vi "Stepper ToGo.vi"(8 "error in":errorcluster, 11 "Arduino Resource":T1={"VISA resource"="", "Board Type"=enum."Arduino Uno", "Connection Type"=enum."USB / Serial", "Bytes Per Packet (15)"=15}) -> (0 "error out":errorcluster, 1 "Steps remaining":u16, 2 "Steps Remaining?":bool, 3 "Arduino Resource Out":T1={"VISA resource"="", "Board Type"=enum."Arduino Uno", "Connection Type"=enum."USB / Serial", "Bytes Per Packet (15)"=15})   [LabVIEW 2011, in "LabVIEW Interface for Arduino.lvlib"]
doc: "Check to see if the Arduino is still processing a previous step command. Wait until Steps Remaining? is false to ensure step commands aren't overwritten."
uses:
  <vilib>/LabVIEW Interface for Arduino/LabVIEW Interface for Arduino.lvlib
  <vilib>/LabVIEW Interface for Arduino/Private/Type Defs/Arduino Resource.ctl
  <vilib>/LabVIEW Interface for Arduino/Private/Type Defs/Board Type.ctl
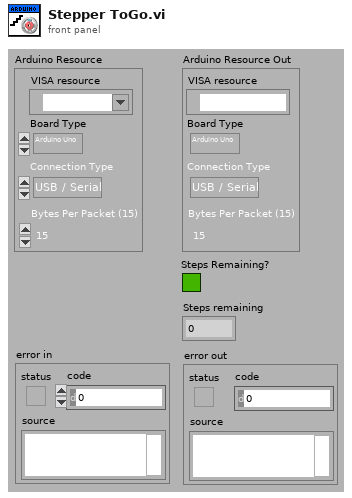
[diagram p1: front panel]
types:
  T1 = typedef "LabVIEW Interface for Arduino.lvlib/Arduino Resource.ctl" = cluster{"VISA resource":refnum<visa-resource-name>, "Board Type":T2, "Connection Type":enum8{"USB / Serial"}, "Bytes Per Packet (15)":u8}
  T2 = typedef "LabVIEW Interface for Arduino.lvlib/Board Type.ctl" = enum16{"Arduino Uno", "Dimuelanove w/Atmega 328", "Mega 2560", "Chipkit Uno32", "Chipkit Max32"}
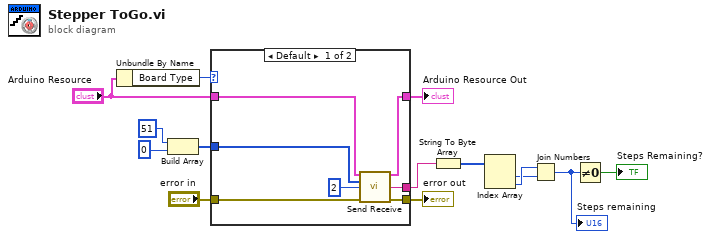
[diagram p0: block diagram]
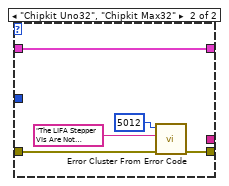
[diagram p2: hidden frame]
diagram:
  n1 = Unbundle By Name("Arduino Resource") -> ("Board Type"=w1:T2)
  n2 = Build Array(u8 51, u8 0 ("element")) -> (w7:u8[])
  n3 = case shown="Default" w1 {
    tunnel: [w19 w24] -> w4
    tunnel: "Arduino Resource" -> [w20 w23]
    tunnel: w7 -> [w18 _]
    tunnel: [w17 w23] -> w6
    tunnel: "error in" -> [w16 w22]
    tunnel: [w15 _] -> w5
    frame Default {
      n4 = call <vilib>:"Send Receive.vi"("Arduino Resource"=w20, "Data"=w18, "Bytes To Read (0)"=u8 2, "error in"=w16) -> ("Arduino Resource"=w17:T1, "Read Buffer"=w15:string, "error out"=w19:errorcluster)  [unwired: 9 in]
    }
    frame "Chipkit Uno32", "Chipkit Max32" {
      n5 = call <vilib>:"Error Cluster From Error Code.vi"("error in (no error)"=w22, "error message (\"\")"="The LIFA Stepper VIs Are Not Supported On Chipkit Targets." ("source"), "error code (0)"=5012) -> ("error out"=w24:errorcluster)  [unwired: 6 in]
    }
  }
  "Arduino Resource Out" <- w6
  "error out" <- w4
  n6 = String To Byte Array(string=w5) -> (unsigned byte array=w13:u8[])
  n7 = Index Array(array=w13) -> (element #1=w10:u8, element #2=w11:u8)  [unwired: 2 in]
  n8 = Join Numbers(hi=w11, lo=w10) -> ((hi.lo)=w8:u16)
  "Steps remaining" <- w8
  n9 = Not Equal To 0?(x=w8) -> (x != 0?=→"Steps Remaining?":bool)
